vi "vector space.vi"(10 "Full transition sequence from service to end":string[](array[string])=["0 1 0", "0 -1 0", "0 2 0", "0 4 0", "-4 1 0", "0 -4 0", "0 -2 0", "1 0 4", "1 -4 0", "0 -3 3", "0 -3 0", "1 -1 0", "-2 2 0", "0 1 -4", "2 0 -3", "0 -3 3 0", "-1 0 -1", "0 -1 1", "2 -1 0", "0 2 -1", "-3 0 1", "0 1 0 4", "1 0 4 0", "-3 3 0", "1 0 -3", "3 -2 0", "2 0 -3 0", "1 0 -1", "-4 0 -1", "0 -4 1", "2 0 -1", "0 -2 2", "-4 0 -3", "0 -1 1 0", "0 2 0 -3", "3 -3 0", "-4 0 1 0", "-4 1 -4 0", "-4 1 0 4", "0 1 -4 0", "-4 1 -4", "0 2 -1 0", "1 0 3", "0 -3 4 0", "-2 0 2", "1 0 1", "4 0 2 0", "0 2 0 3", "0 -1 2", "-1 0 -4", "1 0 -4", "0 -1 0 -1", "-1 0 2", "-1 0 -1 0", "1 0 -2", "0 -4 0 -1", "0 -2 2 0", "-1 0 1", "2 0 2", "0 1 -1 0", "0 3 -3 0", "-4 0 -2", "0 4 -4", "0 -4 0 -3", "0 4 0 1", "0 -2 0 2", "0 4 0 2 0", "-3 0 1 -4 0 -3", "2 0 1 0", "-2 0 2 0", "0 3 -2 0", "-3 3 0 -2 0", "3 -3 0 1", "-3 0 1 0", "4 -4 0", "0 4 -4 0", "0 -3 3 0 -2", "2 0 2 0", "-2 0 -1", "0 -4 0 1 0", "2 0 -4 0", "2 0 -1 0", "-1 3 -2", "2 0 1", "1 0 -3 3 0", "-4 1 -1", "-4 1 -1 0", "-1 0 -3", "3 -2 2", "-1 1 -1 0", "2 0 4", "1 0 -1 0", "0 -1 2 -1", "0 2 0 -2", "-3 0 -4 1", "0 1 0 -1", "-1 3 0", "0 -1 0 -4", "-2 0 -1 0", "4 0 4", "-4 1 0 4 0", "-4 0 -2 0", "-4 0 2", "0 -2 0 2 0", "0 2 0 -4 0", "2 0 4 0", "4 0 -2", "0 1 0 -4 0", "3 0 1", "2 -2 0", "4 0 -2 0", "0 2 0 4", "1 -4 0 1 0", "0 2 0 -2 0", "-2 2 0 -1 0", "-2 2 0 -1", "-1 0 4 0", "-2 0 4", "-4 1 0 3", "0 -3 0 1", "-2 2 0 -3 0", "0 1 0 3", "0 2 0 1", "0 1 0 1 -4", "0 1 -4 1", "-4 1 0 -3", "1 0 -3 0", "-3 0 -2", "2 -1 0 -1 0", "-3 3 0 -2", "1 0 4 -4 0", "0 -4 0 -3 0", "0 -4 0 1 0 -3 3 0", "0 -3 3 0 2 0 -3 0", "0 -3 3 -3 0", "3 -2 0 1", "-4 0 3", "-2 0 1", "0 3 0", "0 -3 4", "-3 4 0", "-3 0 4", "0 3 -3 0 1 -4 0 -3 3", "0 -2 0 -1", "-4 1 0 -2", "-4 0 -2 0 -1", "-2 0 -4", "0 1 0 -2", "0 -1 0 2 0", "0 -2 2 0 -1", "0 -3 -1 3", "-4 -1 0", "0 -1 2 0", "0 -3 0 -4", "2 0 -3 0 -4", "3 0 -1 1", "-4 1 0 -1", "-1 0 -1 2", "-1 0 -4 0", "0 -4 1 -1", "-3 3 -2", "2 -1 1", "4 -3 0", "1 -4 4", "0 2 0 -1", "1 0 1 0", "4 1 0", "0 2 0 2 0", "-4 0 -1 -3", "1 -4 0 -1", "0 -4 1 -4", "-1 3 0 -4 1 -4", "2 -1 3", "1 -3 0", "-2 0 1 -4", "1 0 -1 1", "0 -3 0 -4 1", "0 2 -1 0 1 -4", "0 -1 3", "0 -4 0 -1 0", "0 4 0 -2", "0 -2 0 -1 0", "0 -3 3 0 -2 0", "0 1 -1 0 -1", "0 -1 0 1 -1 0", "-1 3 -2 2", "-2 2 0 1 0 -1", "0 1 -1", "0 4 0 1 0 4", "-3 0 -4", "1 0 4 0 4 0", "4 -4 0 -2", "4 0 2", "-1 2 0", "1 -1 0 -1", "4 0 1", "2 0 3", "0 2 0", "0 -1 0", "0 1 0", "0 3 0", "0 -4 0", "-2 2 0", "1 -1 0", "0 -2 0", "0 -1 2", "0 1 -1", "0 3 -2", "3 -2 0", "0 2 -2", "-1 0 3", "2 -1 0", "-1 0 -1", "-1 0 -3", "-2 2 -2", "2 0 1", "2 0 2", "0 -3 0", "3 -2 2", "0 1 -1 0", "0 -2 2", "-1 2 0", "2 0 -1", "2 -2 0", "3 -3 0", "0 -1 2 0", "0 -1 0 3", "0 -1 1", "0 2 0 1", "2 -2 2", "0 -4 4", "0 4 0", "2 0 3", "-2 3 -2", "2 -2 3", "4 -4 0", "0 1 0 -3", "0 3 0 3", "-1 0 4", "-3 0 -2", "-4 0 -2", "2 0 2 -1", "-1 0 2", "-2 0 -1", "-4 4 0", "0 2 0 -2", "-1 1 -1", "-1 1 -1 0", "-2 0 -2", "3 0 -4 0", "3 0 3", "0 1 0 3", "0 3 -3 0", "2 0 -2", "3 0 -2", "0 -3 3", "3 -2 2 -2", "-3 0 -2 0", "1 0 -3 0", "-1 0 2 0", "3 0 -4", "-1 0 1", "-1 0 -1 0", "0 -1 2 3", "-1 3 -2 0", "3 -1 3", "-2 0 2 0", "0 1 0 -3 0", "0 -4 0 -2", "1 4 -4", "0 -2 2 0", "1 4 0", "0 3 -2 0", "-2 0 -4 4", "-1 0 3 0", "0 2 0 -1", "0 2 -2 3", "4 0 -1", "-1 2 0 2", "1 -1 0 -3", "-2 0 2", "2 0 -4", "0 3 -2 2 -2 2", "0 2 -2 0", "4 0 -4 0", "0 3 0 3 0", "4 -3 0", "-3 4 -3 0", "0 4 -4", "3 0 -1", "-2 2 -2 0", "0 -2 3", "-2 0 3", "1 0 -3", "2 -2 2 0", "0 -3 4", "0 -1 1 -1", "0 4 1 4", "1 -1 0 -1", "1 4 -4 0", "-4 0 2 0", "-4 0 2", "0 -2 2 3 0", "0 -1 1 -1 0", "0 2 0 1 4", "4 0 1 0", "2 3 -2", "0 -1 2 3 -2", "0 -1 0 4", "-4 0 1", "-1 0 -1 2", "-2 0 -1 0", "0 3 0 -1", "3 -2 0 -1", "0 -4 0 -2 0", "2 0 -4 0", "0 -2 0 2", "-1 0 -3 0", "0 -3 0 -2", "2 0 -1 0", "0 -1 2 0 1", "0 -2 0 -4 4 0", "0 -4 4 0", "-1 -3 0", "0 -2 0 3", "2 0 -2 2", "-4 1 0", "-1 1 4", "-1 0 3 -2", "0 2 0 4", "0 -4 4 0 -1", "3 0 -2 0", "0 3 0 -2", "2 0 1 -1 0", "0 1 -1 0 2 0", "0 2 0 1 -1", "2 0 -1 2", "-2 3 0", "0 -1 0 2", "0 1 -1 0 -3", "2 0 1 -1", "-2 0 -1 2", "-1 4 0", "0 -4 1", "2 0 2 0", "2 -1 1", "4 -4 0 -1", "-4 0 -1", "-1 0 4 0", "2 0 2 -1 0", "0 -3 3 0", "-1 0 -3 3", "-1 0 1 -1 0", "0 3 0 -4", "-2 2 -2 0 -2", "-2 0 4 0", "0 1 0 3 0", "4 -3 0 -2 0", "0 3 -2 3", "2 0 3 -2", "3 -2 3", "0 2 -2 3 -2 2", "-2 2 0 3", "3 -2 2 0", "3 -2 2 0 3", "3 -2 3 -2", "0 -3 4 -3 0", "0 -1 0 -3", "3 -3 0 1 0", "0 2 0 3", "0 3 -2 2 -2 2 0", "0 2 0 2", "-2 3 -2 0", "4 0 -2", "-4 0 -1 0 3", "-2 2 -2 3", "0 -1 0 -1 0", "-2 2 0 3 0", "0 2 -2 2", "2 3 -2 2 0", "-2 2 -1", "-4 0 -2 2", "0 -4 0 2", "-1 2 -1", "-1 0 3 -1 3 0 -4", "-1 3 -2", "4 0 -4", "3 0 3 0", "0 3 0", "0 1 0", "0 2 0", "0 4 0", "0 4 -4", "0 -3 4", "0 -3 0", "0 -4 0", "0 3 -2", "0 -1 0", "-4 1 0", "1 0 3", "0 2 0 -3", "2 0 3", "3 -3 0", "-3 0 3", "0 -3 3", "0 -3 4 -3 0", "0 -2 0", "3 -2 0", "0 3 0 1 0", "0 -3 4 0", "2 -2 0", "-2 0 -3", "4 0 2", "-3 0 2", "0 3 -3 0", "4 -4 0", "0 -1 2", "3 0 4", "0 3 -2 0", "0 -3 0 3", "1 0 -1", "0 4 -4 0", "-2 0 3", "0 2 -2 0", "0 2 0 -3 4", "3 -3 0 -3", "4 0 2 0", "3 0 -2", "0 -3 3 0", "-1 0 3", "0 -1 2 0", "-4 0 -1", "2 0 3 0", "0 3 0 3", "-4 0 3", "0 4 -4 1", "4 0 -3", "0 -1 0 4", "0 3 -3 0 2", "0 -2 0 3", "0 -3 4 0 3 0", "-3 0 4 0", "0 3 0 3 0", "0 4 0 -3 0", "-3 4 0", "2 0 -3 4", "0 2 0 -3 4 0", "0 1 0 2", "0 -2 3", "-2 0 -2", "0 -3 4 0 2", "0 -3 3 0 -2 2", "1 0 -3", "0 -1 1 0", "4 -4 0 -4", "-4 0 3 0", "2 0 -3", "-2 0 3 0", "0 4 -4 1 0", "-4 1 0 -1 2 0", "3 0 4 -4", "0 -3 4 -3 0 2", "3 0 3", "-1 0 -3", "-3 4 -3", "4 -3 0", "0 -3 4 -3", "-3 4 -3 0", "4 0 2 0 3", "0 2 0 3", "-4 1 0 -4 0 4 -4", "-4 1 -1", "-1 0 -4 0", "1 0 3 -2", "0 -1 0 3", "0 3 0 4 0", "0 2 0 3 0 1 0", "-4 1 -4 1", "1 -4 1 0", "0 -4 4", "0 1 0 4", "1 -4 1", "-3 0 1", "0 4 -4 0 -1 0", "-3 0 4", "2 0 -3 4 0", "1 0 2", "4 -3 0 2", "-3 4 -3 0 2", "3 0 1", "1 -1 0", "0 -1 0", "0 1 0", "0 1 -1 0", "0 4 0", "0 3 0", "-1 0 4", "-1 0 -3 3", "1 0 1", "-4 1 -1", "0 4 0 2", "0 -1 0 -3", "3 -2 2 -1 0", "2 -1 0", "0 1 -1", "-1 0 3", "-1 1 -1 0", "-3 0 1", "-1 0 3 0 -4", "-1 0 -3", "1 -1 0 -3 3", "1 -1 0 3", "2 -1 0 4 -4", "1 0 1 0", "0 -1 0 4", "2 0 3 0 -1", "-4 1 -1 0", "0 3 0", "0 -1 0", "0 4 0", "-1 0 3", "0 -3 4", "0 -3 3", "1 -1 0", "0 3 -2", "0 2 0", "0 1 -1", "4 -3 0", "-4 0 -3", "0 -4 0", "4 0 2", "0 1 -1 0", "0 1 0", "0 4 -4", "3 -2 2", "2 -1 0", "0 -2 0", "0 -3 4 0", "-1 0 -3", "0 3 -2 0", "0 -3 3 -3 0", "0 -3 4 -3 0", "4 0 4", "0 1 -1 0 3", "3 -2 2 0", "-2 2 0", "3 0 1", "0 4 0 2", "0 2 -1", "2 0 4", "-1 0 4", "0 -3 3 0", "-1 0 1", "-1 0 -1 0", "-1 0 -1", "4 -3 0 2", "0 -3 0", "-4 0 -3 0", "-3 0 3 -2", "0 3 -2 2 0", "-4 0 -3 3", "0 3 0 -4", "2 0 4 -4", "0 2 0 4", "0 4 0 -4", "2 -1 0 1 -1 0", "0 2 -1 0", "-1 0 -3 3", "0 -4 4 0", "0 4 -4 0", "-4 0 3 0", "0 -2 3", "-3 0 -3", "0 -2 0 -3", "-3 0 1", "-2 3 0", "0 3 0 -2", "0 4 -3 0", "4 -3 0 2 0", "0 -3 4 -3 0 3 -2 2 0", "3 0 -3 4 -3 0", "-1 0 3 -2 3", "-1 0 3 -2", "0 1 0 3", "1 0 3", "4 -3 0 -2", "-4 0 -3 4", "-2 0 3 0", "2 0 2", "0 2 0 2 0", "-4 4 -3 0", "0 -4 0 -3", "3 0 3 0", "-4 0 -3 3 0", "4 0 3", "0 4 0 4", "4 0 4 0", "0 4 0 -4 0", "0 -1 0 -2", "4 0 2 0", "1 0 -3", "0 -4 1 -4", "0 4 -4 0 -3", "-2 2 0 4 -4", "0 4 -4 4 -4", "4 0 2 -2", "0 4 0 -2", "0 3 0 1", "4 -4 1", "4 0 2 -1 0", "0 -4 4 0 2", "-1 0 3 0", "0 3 -2 0 -1 0", "1 -1 0 4", "0 4 0 1", "-1 0 4 0", "1 0 3 -2 0 -1 0", "0 -4 0 3 0 -4", "-1 0 -4", "1 -4 0", "1 0 4 0", "0 -1 0 -1 0", "-1 0 -3 3 0", "0 -1 0 -1 0 -3", "-2 2 -1 0", "0 -1 0 3 -2", "2 -1 0 1 -1 0 3", "-2 3 -2 2 -1", "-2 2 -1", "0 -1 0 4", "3 0 1 0", "0 3 -2 0 -1 0 -1 0", "-3 4 0", "3 0 -1", "0 4 -3", "3 0 3", "-4 0 3", "4 -4 0", "0 -1 0 -1", "0 3 0", "0 -3 4", "0 -3 3", "0 3 -3 0", "0 2 0", "4 -3 0", "0 3 -3", "0 3 -2", "0 -3 4 -3 0", "-4 0 -3", "3 0 -3", "0 -4 0", "-3 0 -3", "0 -3 3 0 3", "0 -3 3 0", "0 -2 0", "-3 0 3", "3 -3 0", "3 0 3", "-3 4 0", "-4 0 -3 4", "-3 0 4", "0 -1 0", "3 0 -3 3", "-3 3 0", "0 3 -2 0", "0 -3 4 0", "1 0 -3 4", "0 -3 0", "0 -1 0 -3", "-3 0 3 0", "-2 0 3 -2", "0 1 0", "0 -2 0 3", "-2 0 -3", "0 3 0 -3", "3 0 3 -3", "3 -3 0 3", "-3 0 -3 3 0", "0 -3 4 -4 0", "0 2 0 -2", "-2 0 3", "0 3 -2 3 0", "-2 3 0 -3 3", "3 0 -1", "-3 0 -4", "1 -1 0", "-4 0 -2", "0 3 -3 0 4", "-2 3 0", "-1 0 3 -2", "-3 4 -3", "0 -3 4 -3", "-3 4 -3 0", "-3 3 0 3", "-2 0 2", "0 -1 0", "0 -2 3", "3 -2 0", "-2 3 -2 0", "0 2 0", "0 1 0", "0 4 0", "2 0 -1 0", "0 3 -2", "2 -2 3", "-2 0 2", "0 2 -2 0", "4 -3 0", "-3 0 -2 0", "0 3 0", "0 -3 -2", "-2 3 -2 0 3", "0 3 0", "0 -2 0", "0 1 0", "0 3 -2", "2 -2 0", "0 2 0", "3 -2 0", "0 -3 4", "0 4 0", "-2 0 -2", "0 -3 0", "3 -2 2", "1 -1 0", "0 2 -2", "-2 3 -2", "0 -1 0", "0 -4 0", "0 2 -2 0", "-1 0 3", "0 -2 3", "2 0 -2", "0 3 -2 0", "0 -3 4 0", "-3 0 3", "0 3 -3", "4 -3 0", "-2 0 -3", "0 -2 3 -2", "-2 2 0", "0 3 -2 2", "3 -2 2 0", "2 0 2", "3 -3 0", "2 0 3", "0 -2 0 -2", "-3 4 0", "0 3 -3 0", "-1 0 3 0", "-2 0 1", "2 -1 0", "0 -3 4 -3", "0 3 -2 2 0", "-2 0 1 0", "-3 0 4", "0 -2 2", "-2 3 -2 0", "0 3 -2 3", "0 1 -1 0", "1 0 1", "0 -3 0 3", "0 -3 3", "3 0 -3", "0 -1 0 3", "4 0 1 0", "0 -2 3 -2 0", "2 0 3 -2 0", "0 2 -1", "3 -3 0 4 0", "-2 0 -4", "-3 0 -2", "3 0 3", "0 3 0 3 0", "0 3 -2 3 -2", "-2 3 -2 2", "-3 0 1", "-2 0 3", "-2 0 -3 0", "0 3 -2 2 0 2", "2 0 2 0", "1 -1 0 3", "0 3 -2 0 -2 2", "-2 0 -2 2", "2 0 -2 3 -2", "1 0 -2", "1 0 3", "2 0 -4 0", "-1 0 1", "0 2 0 4", "4 0 -2", "0 -2 0 1", "0 -1 0 3 0", "0 2 0 3 -2 0", "0 3 -2 0 1 0", "-1 0 -1 0", "-2 2 0 -2", "2 0 -2 0 -2", "0 4 0 1 0", "0 1 0 4 0", "0 1 0 -3", "0 -3 0 3 -2", "1 0 -3 0", "4 0 -4 0 1", "-1 0 -4", "0 -3 3 -3 0 4 0", "0 -4 0 3", "0 3 0 2", "1 0 1 0", "0 4 0 3", "1 -1 0 -3 4 0", "3 -2 0 -4", "2 -1 2 0", "-4 1 0", "3 -2 0 -4 0", "-2 0 -3 4", "0 -3 4 -3 0", "0 -2 0 -3", "-2 0 -3 4 -3 0", "2 -2 3", "0 2 -1 0", "2 0 2 -2 0", "0 -3 4 0 2", "1 0 2", "-3 4 0 2 0", "-2 0 -4 1", "0 3 -2 0 -4", "0 2 0 2", "-2 3 0", "1 0 -3", "0 3 0 -3 4", "-3 4 0 2", "-2 0 -2 2 -2 0", "2 -2 0 -3 4", "0 -3 4 -3 0 3", "4 -3 0 3 0", "3 0 -2", "0 -2 0 -2 0", "4 -3 0 3", "0 4 -3 0", "-3 0 -2 0", "-1 0 -1", "1 0 4", "2 0 2 -2", "-2 0 -2 0", "1 -1 0", "-1 0 1", "0 1 0", "0 -1 0", "0 1 -1", "-1 0 -1", "0 4 0", "2 -1 0", "-1 0 1 -1", "-1 0 4", "0 -3 0", "0 1 -1 0", "-1 1 -1", "-1 0 -3", "-1 0 -1 0", "0 -1 0 1", "1 -1 0 -1", "-1 1 -1 0", "1 -1 1", "4 0 2", "0 1 -1 0 1", "1 -1 0 4", "0 1 0 -4", "0 4 -4", "-1 0 -1 0 1", "-1 0 4 0", "0 1 -1 1 -1 0", "1 0 -4 0", "1 0 -4", "0 4 0 -1 0", "-1 0 1 0", "0 4 -4 0", "-1 0 -3 4 0", "0 1 0 -1 0 -3", "0 1 0 -4 0", "-4 0 4", "0 -1 1 -1", "-2 2 -1 0", "0 -3 0 -1 0", "2 -1 0 -3", "-1 0 3 0", "-1 0 -3 0", "-1 0 -2", "0 2 0", "1 -1 0 4 0", "-1 0 4 0 -1 0", "0 1 -1 1 -1 0 4", "0 -2 2 -2", "-1 0 -1 0 1 0", "3 0 1 0", "0 4 0 1 -1", "1 -1 0 1", "0 1 -1 1", "1 -1 1 -1", "0 1 -1 1 -1", "1 -1 1 -1 0", "0 -1 1", "0 -4 0", "-3 0 -1", "4 0 -1", "-1 1 -1 0 4", "1 -1 1 -1 0 4", "-2 2 0", "1 -1 0", "0 1 0", "0 -1 0", "3 -3 0", "0 3 0", "0 1 -1", "0 4 0", "0 2 0", "2 -1 0", "-1 0 1", "0 -2 0", "-4 1 0", "1 0 1", "0 1 -1 0", "-1 0 -3", "-1 0 4", "0 4 0 -2", "0 4 -4", "-1 0 1 0", "0 3 -3 0", "0 -4 1", "0 4 -4 1", "-4 4 0", "-1 0 3", "0 -2 3", "0 -3 4", "1 0 1 -1", "-2 0 -3", "0 -3 0", "0 -3 3", "-2 3 -3 0", "1 0 -2", "-2 3 -2", "4 -4 1", "1 -1 0 4 -4 1", "-1 0 4 -4 1 -1", "-4 1 0 1 -1 0", "0 1 0 -4", "0 1 0 -2", "-1 0 -1 0", "2 -1 0 1", "1 -1 0 1 0", "3 -2 0", "0 -2 2", "2 0 2", "3 -3 0 1", "-3 0 3", "-2 2 0 -3", "0 3 -3", "-3 0 -4 4", "0 4 0 -2 3", "0 -4 4", "-1 0 3 0", "4 -4 1 0 4", "4 0 1 0", "1 -1 0 -3", "-2 0 1 -1", "0 4 -4 1 0", "0 -4 4 0 1", "1 0 -2 3 -2", "1 0 4", "0 -4 1 0", "0 1 0 -4 1 0", "-2 0 1", "4 -3 0", "-3 0 4", "0 4 -3 0", "1 -1 0 4 -4 1 -1 0", "4 -4 1 0", "1 0 4 0", "1 -1 0 -1 0", "0 -4 0", "4 0 1", "0 1 0 1 0", "2 0 4 0", "0 -2 0 2 0", "2 0 1", "-1 0 -3 4", "4 0 2 0", "0 -2 0 1", "-1 0 4 -4 1", "3 -2 3", "3 -2 2 0", "1 -1 0 3", "-1 0 -1", "0 -1 1", "-1 0 1 0 3", "0 -4 1 0 1 -1 0", "0 3 -2", "0 1 0 3", "1 -4 0", "0 -2 2 0", "1 -1 1 -1 0", "0 1 0 3 -3 0", "-3 0 -3 3", "0 -3 3 0", "0 3 0 -2 0", "0 2 0 2", "-4 0 -2", "3 0 3", "3 0 3 0", "0 -3 3 -2", "0 2 -2 3 -3 0", "-2 2 0 -3 3", "-3 0 1", "3 -3 0 3", "0 3 -3 0 1", "0 3 0 2", "2 0 -3", "-2 3 -3", "3 -2 2", "-4 1 -1", "2 0 -3 3", "0 4 0", "0 -2 0", "1 -1 0", "-1 2 -1", "0 2 0", "2 -1 0", "0 3 0", "0 -1 0", "-2 0 3", "0 -4 0", "3 -2 0", "0 3 -2", "0 -3 0", "-1 0 3", "0 -2 0 3", "0 1 -1 0", "0 3 -2 0", "1 -4 0", "-1 0 2", "0 -1 2", "2 0 3", "0 -3 3", "3 -3 0", "3 0 -1 0", "-2 0 -2", "2 -2 0", "-3 3 0", "0 2 0 3", "0 1 0", "0 -2 2", "-4 0 -1", "0 -1 2 -1", "-1 0 -1", "2 -1 2", "-1 3 -2", "3 0 -4", "3 -2 2", "-1 1 -1 0", "-1 2 -1 0", "0 1 -4", "4 -4 0", "2 -3 0", "0 3 0 -2", "2 0 3 0", "0 1 0 -3", "1 0 -3", "-1 0 -4 0", "-4 0 1", "2 0 -2 0", "-1 0 -3", "0 -3 4", "4 0 1", "0 1 -4 0", "0 -1 0 3", "0 -3 3 0", "0 3 -3 0", "0 4 0 2", "0 2 -2 0", "-2 0 -3", "3 0 3", "-1 0 -2", "-2 0 3 0", "2 0 4 0", "0 4 0 -2 3", "0 -3 0 -2", "-3 0 -2 2", "1 0 4 0", "-3 0 2", "0 -2 0 3 -2 0", "1 0 -3 0", "-3 0 -2", "-2 0 -2 0", "0 4 -4", "-1 -3 0", "-2 2 -1", "2 0 -3", "-1 1 0", "2 -1 1", "-2 2 0", "0 -4 0 -1", "0 -1 3 -2 2", "-1 2 -1 2", "-1 2 0", "-1 3 0 -1 0", "2 0 2", "-1 0 2 -3 0", "-1 0 2 0", "-1 4 -4 1", "-1 0 4", "2 -1 0 -1", "2 -1 0 2", "-4 1 -1", "3 0 -4 1", "1 -1 -3 3", "0 1 0", "0 -2 0", "1 -1 0", "0 3 0", "0 2 0", "0 3 -2", "3 -2 0", "0 -4 0", "-1 0 -2", "-2 2 0", "0 -1 0", "1 -1 0 -2", "0 -2 2", "-2 0 -2", "0 1 0 1", "4 -4 0", "0 3 -3", "0 1 -1", "1 0 1", "0 3 -2 0", "-2 2 -2", "0 -2 3", "0 3 -3 0", "0 4 0", "2 0 3", "0 -2 3 -2", "0 4 -4 0", "-2 0 -2 0", "1 -1 0 -2 0", "-2 0 2", "-4 0 -4", "0 -4 0 1", "0 2 0 -4", "3 0 -2", "-1 0 3", "0 1 -1 0", "-3 0 -1", "-1 0 2 0", "4 -3 0", "1 0 -2", "0 1 0 1 0", "0 -2 3 -2 0", "3 -2 0 -2 0", "0 -2 2 -2 0", "0 -2 0 -2", "-1 4 0", "4 0 2", "1 -1 0 -2 0 2 0", "2 0 -2", "-2 0 4", "0 -1 0 3", "0 -2 2 0", "1 0 3", "0 1 0 3", "4 0 -2", "0 -4 0 -4", "0 2 0 -4 0", "-4 0 -4 0 1 0", "-1 2 3 0", "3 0 3", "0 -4 0 3 0", "2 0 1", "2 -1 0", "-1 0 -1", "-2 3 0 -2", "3 0 -2 0", "0 1 -1 0 -2", "0 3 0 -2", "3 -2 2 -2", "1 0 1 -1", "0 4 -3 0", "2 0 -1 0", "0 2 0 3", "2 0 3 0", "2 0 -3 4 -3", "-2 2 0 -3 4", "2 0 -3 4", "0 3 -3 0 -1 0", "1 0 4", "0 3 0 1", "1 0 3 -2 0", "-2 3 0", "1 0 1 0", "0 4 0", "0 2 0", "0 3 0", "0 -3 0", "0 1 0", "-4 0 -3", "0 -4 0", "0 3 -3 0", "0 -3 0 3", "-4 0 3", "0 4 0 2", "0 -3 3", "-4 0 -3 0 3", "0 2 0 3", "-3 0 2", "0 4 0 1", "0 -4 0 3", "0 4 0 2 0", "0 -2 0", "0 1 0 4", "4 0 2", "0 4 0", "0 3 0", "0 2 0", "4 -4 0", "0 4 -4 0", "0 -2 0", "3 -3 0", "0 4 -4", "0 3 -3", "0 3 -2", "0 4 0 2", "4 0 2", "0 1 0", "0 3 -3 0", "0 -3 0", "2 -1 0", "0 -1 0", "1 0 3", "4 0 3", "3 -2 0", "0 1 -4", "-1 0 4", "0 -4 0", "0 -3 3", "2 0 4", "-4 1 0", "0 -2 2", "0 4 0 3", "-1 0 1", "0 3 -2 0", "-3 0 4", "-1 0 3", "0 -3 4", "0 4 0 -2", "1 -1 0", "2 0 4 0", "0 -4 4", "0 -1 0 4", "-1 0 4 0", "4 -3 0", "0 2 -1 0", "1 -4 0", "2 0 -4", "-2 0 4", "0 4 0 2 0", "3 0 3", "0 -3 3 0", "2 -2 0", "1 0 -3", "-4 0 2", "1 0 3 0", "0 1 0 3", "-1 0 3 0", "3 -2 2", "-4 1 -1", "2 0 -3", "0 -4 1", "0 2 0 -4", "-3 0 4 0", "3 0 -2", "0 -2 2 0", "0 -2 3", "-4 0 2 0", "0 3 0 -4", "0 2 0 4 0", "-2 0 2", "-2 2 0", "0 3 0 4", "-3 4 0", "-1 0 1 0", "4 0 4", "0 1 0 3 0", "0 -1 0 4 0", "0 3 0 3", "1 0 -3 0", "0 3 0 1", "-2 2 -1 0", "0 3 -2 2", "-3 0 2", "1 -1 0 3 0", "0 3 0 -2", "-4 0 -4", "0 1 0 -3 0", "0 4 0 -3", "2 -1 0 4", "1 -4 1", "-4 0 3", "-2 0 -4 0", "0 3 -3 0 4", "-4 0 -2", "0 4 -4 0 3", "0 -2 3 -2 0", "0 4 0 4", "-1 2 -1", "-3 0 -2", "-3 0 -3", "-4 0 4", "4 0 -3", "3 0 -4", "2 0 -2", "-2 0 2 0", "0 -4 4 0", "0 2 0 3", "-2 0 1", "4 0 3 -3 0", "0 -2 0 3", "0 4 0 3 0", "0 2 -2 0", "2 -2 0 4", "4 0 -2", "2 0 -1", "0 1 -4 0", "0 -1 2", "4 0 -1", "0 1 -4 1", "4 -4 1", "0 3 -2 0 1", "4 0 4 0", "0 -1 0 4 0 4", "1 0 4", "0 1 -4 1 0", "0 4 0 2 0 -3", "-2 0 4 0", "0 2 -2 0 4 0", "0 -3 0 2", "-4 0 -2 0", "0 -2 0 2 0", "0 2 0 -1", "0 -1 3", "0 -4 4 -4", "3 -2 0 -4 0", "-4 0 -1", "-3 0 3 0 3", "-1 0 3 -3 0", "-3 0 3 0", "0 3 0 3 -2", "-2 2 -2", "-1 0 1 0 3", "-2 2 -1 0 1 0", "0 2 -1 0 -3", "0 4 0 2 -1 0", "-1 0 4 -4 0", "0 2 -1 0 4 -4", "0 4 -4 0 3 -2 0", "-1 0 -3", "-2 0 1 -4", "0 3 0 4 0", "0 1 -4 4", "-1 0 -3 0", "-1 0 4 -4", "0 4 0 -2 0", "0 4 -3 0", "4 0 -3 3", "-1 0 -2", "0 -2 0 3 -3", "1 -4 1 -1 0", "-4 1 -1 0", "-2 0 -2 2", "0 -1 2 -1", "-4 0 -4 1", "0 2 0 4 0 2 0", "0 3 0 -1", "3 0 3 0", "0 -3 0 3 0", "0 3 0 4 -4 1", "-1 0 -4", "0 -4 1 0 3 0", "0 2 -1", "-4 0 4 0", "0 -2 0 4", "0 4 0 -1", "-4 0 3 0", "0 3 0 -2 0", "0 -3 4 -3 0", "-4 0 2 0 -4", "2 0 -2 0", "-2 2 0 -3", "3 0 2 0 4 0", "3 0 2 0", "1 -4 0 2 0", "3 0 -4 4 0", "3 0 -4 4", "3 -3 0 4", "-2 3 -3", "0 -4 0 2 0", "0 3 0 -4 0", "3 -3 0 4 0", "0 3 -3 0 4 0", "4 0 3 -2", "-4 0 -3", "-3 0 -3 4", "3 -3 4 0", "1 -4 -1", "-3 3 -3 0", "0 -1 1", "-3 0 4 0 3", "0 3 -3 0 -2", "0 4 0 3 -3 0", "4 -3 0 4", "0 3 0 2 0", "0 4 0 -2 2", "-4 -1 0 1", "-1 0 1 0 -3 0", "-3 0 1 -4 0", "-3 3 0", "0 -1 0 1", "-1 0 1 -4", "0 3 0 -4 4", "-4 1 -1 0 3 0", "0 1 0 3 0 1", "-3 0 3", "4 0 -2 0", "4 0 2 0", "3 0 -1", "4 0 3 -3", "3 -3 0 -2", "3 0 4", "3 0 2", "2 0 3", "4 0 -2 2", "-2 2 -1", "0 2 -1", "0 4 0", "2 -1 0", "0 -4 0", "0 2 -1 0", "3 -2 0", "4 -3 0", "0 -1 2 0", "0 -1 0", "0 2 -2", "-4 0 1", "-4 0 -4", "0 -4 0 -4 0", "-1 0 4 0 2", "-2 2 0", "1 0 -4 0", "3 -2 2", "0 2 3 -2", "2 -1 0 2 -1", "2 -1 -3", "3 -2 0 -4", "0 -3 4 -3 0", "-1 1 -1 0 -1", "0 -4 1 0", "-1 0 2", "4 0 2", "0 2 0", "0 1 0", "0 -4 0", "0 -2 0", "0 2 -2", "2 -2 0", "0 4 0", "0 3 0", "0 2 -2 0", "0 -1 0", "0 -3 0", "-4 0 -2", "-2 0 2", "1 0 4", "-2 0 -4", "0 3 -2", "3 -2 0", "1 -1 0", "-2 3 0", "0 -1 2", "0 -3 4", "4 -3 0", "-2 0 4", "0 4 -3", "-2 0 -4 0", "-2 2 -2", "3 0 1", "4 0 2", "-1 0 -1", "0 -2 3", "1 0 -4", "-1 0 -1 0", "-2 0 -3", "1 0 -3", "-2 0 3", "2 0 -2", "-2 2 -2 0", "-4 0 -2 0", "0 1 0 4", "0 3 -3", "2 0 1", "1 -4 0", "0 -4 1", "0 3 -2 0", "-3 4 0", "0 -4 0 -2", "2 -1 0", "0 3 0 1", "0 1 -4 0", "3 0 2", "-3 0 -4", "-4 0 2 -2 0", "0 -4 0 2 -2", "2 0 -2 0", "0 4 -3 0", "-4 0 2", "-4 0 2 -2", "-2 2 0", "-4 1 0", "0 4 -4", "-2 0 2 0", "0 -2 0 2", "1 0 3", "-2 0 4 0", "2 0 -4", "-2 3 -2", "0 2 0 1", "0 4 0 2", "0 2 -2 2", "0 1 -1", "0 -4 0 -3", "-1 0 -4", "-1 0 -2", "2 -2 0 -4 0", "2 0 3", "0 -4 0 2", "0 -3 4 0", "0 3 -3 0", "0 -4 0 -2 0", "-2 0 -2", "0 -3 3", "0 -2 0 -4", "0 -4 1 0", "4 0 2 -2", "-3 0 -4 0", "0 -3 4 -3 0", "2 -2 0 2", "0 1 0 -1", "2 -2 0 4 0", "2 -2 0 4", "1 0 -4 0", "-3 0 3 0", "0 3 0 -2", "2 -2 3", "0 2 0 -2 0", "0 1 0 3", "1 0 4 0", "-4 4 -4 0", "-2 0 1", "0 -4 0 3 0", "1 0 1 0", "-1 0 3", "0 -1 2 -1", "0 -1 0 -1", "0 4 0 3", "0 -2 0 4", "0 -4 4", "0 3 0 1 0", "1 0 -3 3", "0 2 -1", "-1 0 1", "-2 0 -3 0", "1 -1 0 -2", "-1 0 -2 0", "3 0 3", "-1 1 0", "3 0 -2", "3 0 4 0", "0 2 -2 2 -2 0", "0 1 0 -4", "0 2 0 4 -3", "-2 0 -2 0", "0 3 0 -2 0", "-2 0 -2 3", "0 2 0 3", "0 -2 0 2 0", "0 -3 3 0", "4 0 -3", "0 1 0 -3", "1 0 4 -3 0", "2 -2 0 -2", "0 -1 1", "-1 1 -1 0", "0 1 0 -1 1", "0 -3 0 -3", "-1 0 -3", "4 -3 0 1", "-3 4 0 2", "0 2 -2 0 -3 4", "3 -2 0 -3 0", "0 -2 0 3", "-2 0 -4 0 2", "0 2 -2 0 -4 0", "0 -2 0 4 0 3", "4 0 -2 0", "0 -4 0 -3 4", "0 1 0 -4 0", "0 -2 2", "0 4 0 4", "2 0 -4 0", "-4 0 -1 2", "3 0 3 0", "0 3 0 2", "0 2 -1 0", "2 -2 3 0", "0 1 -1 0", "0 1 0 4 0", "0 1 -4 0 -2", "0 -2 0 2 -2 0", "0 -2 0 -3", "-4 0 1", "-2 0 2 -2 0 3 0", "-2 0 3 0 1 -4 0", "4 -1 0", "0 2 -2 0 2", "2 0 2 -2", "1 0 -4 4", "-1 0 4", "2 -1 0 -4 0 -3", "0 -1 2 -1 0", "-1 0 3 0", "-3 0 3 0 1 0", "1 -4 0 -4", "0 1 0 -2", "-2 0 -4 0 3 0", "0 4 0 2 -2 2 -2 0 -4 0 3", "0 2 -2 0 4", "-2 0 2 -2 0", "0 -1 1 0", "1 -1 0 -2 0", "0 -4 0 3", "4 0 1", "-2 0 -1", "-1 0 -1 0 -1", "0 1 0 3 0", "-1 2 0", "-1 0 1 0", "3 -2 3", "0 -2 3 0", "3 0 2 0", "0 3 0 4 0", "-1 0 2", "0 -3 0 -1 0", "-4 0 -3", "-1 0 -2 3", "0 -2 3 -2", "0 -2 3 -2 0", "-2 0 -4 0 3", "0 3 0 3", "0 -2 0 -4 0", "0 4 0 -4 0", "1 0 2", "3 0 -2 3 -2", "-3 0 2 -2 0", "4 -3 0 2", "-3 0 -2 0", "2 0 4", "0 2 0 4", "2 0 4 -3", "0 2 0 4 -3 0", "-3 0 2", "-3 0 -3", "4 0 4", "1 0 -2", "-2 0 2 -2", "1 0 1", "2 0 4 -3 0", "-3 0 3", "3 -3 0", "0 3 0", "-3 3 -3 0", "-3 3 -3", "0 -3 3 -3", "0 -3 3 -3 0", "2 -1 0", "0 -3 3", "-3 0 -3", "3 -3 0 -3", "-3 0 -3 3", "0 2 -1", "0 1 0", "0 3 0 3", "0 -1 0", "3 -3 0 -3 3", "0 2 -1 0", "0 4 0", "0 3 -2", "-1 0 2", "3 -2 0", "0 -4 0", "0 -3 0", "3 0 2", "0 3 -3", "0 -3 4", "-3 0 -3 3 -3", "0 3 -2 0", "-1 0 4", "-1 0 3", "-1 0 3 0", "0 1 0 3 0", "1 0 -1", "0 1 0 -1 0", "3 0 1", "0 2 0", "0 -1 2 0", "-3 0 -2", "3 0 -3", "0 -2 3", "0 -3 3 -3 0 -3 3", "3 0 3", "0 2 -1 0 2", "0 2 -2", "2 -2 3", "1 -1 0 3", "0 3 -2 0 1 0", "0 4 0 -1", "0 1 -4", "2 -1 0 4", "0 4 -4", "0 1 0 3 0 1 0", "1 0 3", "0 1 0 3", "1 0 3 0", "2 0 -1", "0 -1 0 3 0 3 0", "0 2 0 3 0", "2 0 4 0 2", "-4 0 -3", "4 -4 0", "0 3 0 3 -3", "-4 0 3 0", "0 -3 4 -3", "-3 3 0", "-2 0 3", "0 -2 0", "1 0 -3", "2 -2 0", "3 0 -3 4", "-3 0 -3 3 -3 0", "3 -3 0 -3 3 -3 0", "0 -3 3 -3 0 -3 3 -3 0", "0 3 0 -3", "-3 3 -3 0 -3", "0 -3 3 -3 0 -3", "-3 3 -3 0 -3 3", "2 -1 0 2", "3 0 3 0", "2 0 3", "3 -3 0 -3 3 -3", "0 3 0", "0 2 0", "0 4 0", "0 -3 4", "0 1 0", "2 -1 0", "0 -1 0", "0 -3 3", "2 0 3", "0 4 -4", "1 -1 0", "0 3 -2", "3 0 3", "0 2 -1", "-4 0 -3", "0 -3 0", "-1 0 4", "-1 0 2", "4 -4 1", "4 -4 0", "0 -2 3", "3 -3 0", "0 1 -1", "0 1 -4 0", "3 0 3 0", "1 -4 0", "0 2 0 3", "3 -2 0", "0 3 0 3", "-1 0 3", "1 -1 0 4", "0 2 -1 0", "0 -3 4 -4", "3 0 1", "0 -2 0", "0 4 -4 0", "0 3 0 3 0", "1 0 3 0", "3 -2 2", "-4 0 -3 3", "3 0 -3", "0 -3 3 -3 0", "3 0 -2", "-4 1 0", "0 -4 4", "2 -1 0 -3", "0 3 0 1", "2 0 -3", "-3 0 1", "-4 1 -1", "0 2 -2", "-2 3 0", "1 0 1", "0 -1 0 2", "0 3 -2 2", "0 1 0 3", "0 -4 1", "0 -3 3 0", "-2 2 0", "-2 0 3", "1 0 4 0", "4 -4 1 0", "0 1 -1 2", "1 0 1 0", "0 1 0 1", "-1 0 4 -4", "2 -1 0 3", "1 -1 2", "-1 2 -1 0", "0 4 -4 1 -1", "0 -3 4 -4 1", "4 -4 0 -3 3", "0 -4 4 -4", "-1 0 2 -1", "-2 0 -1", "1 -1 0 4 -4", "0 4 0 3", "2 0 4", "4 -4 0 -3", "0 3 0 -2", "0 -3 4 0", "1 0 3", "-4 0 3", "-3 0 2", "0 3 -2 3", "0 2 0 3 0", "0 4 0 2", "4 -3 0", "-3 0 1 0", "0 2 0 -3", "0 1 0 3 0", "0 -4 0", "0 -4 0 -3", "2 -2 0", "2 0 -2", "0 3 -3", "2 -1 0 -3 4", "-1 0 -2", "1 -1 0 3", "-1 0 3 0", "0 -1 2", "0 -3 4 -4 1 0", "0 4 0 -1", "1 0 -3", "0 3 -2 0", "0 1 0 4 0", "0 4 0 -4", "0 4 0 3 -2", "3 -2 0 1 0", "2 -1 0 -3 0", "-3 0 -4", "0 4 -4 1 -1 0", "-1 0 4 -4 0", "0 4 -4 0 2", "-3 0 -1", "0 3 0 1 -1", "-1 0 4 0", "0 1 -1 2 -1 0", "2 -1 0 2", "0 2 0 -1", "-1 0 -1 0", "-1 0 2 -1 0", "0 1 0 2", "0 2 0 -3 4 -4", "1 0 3 0 2", "0 -2 3 -2", "3 -2 0 -1", "0 4 -4 0 -3", "1 0 -4", "-4 0 -3 3 -3 0", "-2 3 -2 0", "-2 3 -2", "0 4 0 2 0", "-4 0 3 0", "0 1 -4", "0 -3 3 0 -2", "0 -2 0 2", "-2 0 2 0", "3 0 -2 0", "-4 0 -3 0", "0 -3 0 3", "0 3 -3 0", "0 -3 4 -3 0 1 0", "0 3 -2 2 0", "2 0 2", "0 2 0 2 0", "0 3 0 -3", "3 0 -3 4", "0 1 0 1 0", "0 -3 3 -2 0 3", "0 -3 4 -4 0 -3 3 -2", "0 -3 0 2 0", "0 2 -2 0", "0 -3 3 -2", "2 0 -4 0 -3 3", "3 0 -2 3", "0 2 0 -2", "0 2 0 4 0", "-2 0 -2 3 0", "0 1 0 3 0 -2", "-3 3 -3", "0 -3 3 -3", "-3 3 -3 0", "1 0 4", "-4 0 2", "-1 0 -1", "3 0 2", "-3 4 -4", "4 0 3", "-2 0 2", "2 0 3 0", "0 2 -1 0 3", "-3 3 -2", "0 -1 0", "0 3 0", "-1 0 3", "0 3 -2", "-1 0 3 0", "0 1 0", "0 3 0 -1", "-1 0 -1", "3 0 -1", "0 -1 0 3", "-1 1 0", "-1 0 3 -2", "-1 0 -1 0", "0 -1 1 0", "0 -1 0 -1", "0 -1 1", "3 -3 0", "0 1 -1", "0 3 -3", "0 -1 0 -1 0", "0 -3 3", "0 -3 3 0", "0 3 0 3", "1 0 -1", "0 1 -1 0 3", "0 3 0 -1 1 0", "2 -1 0", "1 0 3", "0 3 -2 0", "0 3 -3 0", "0 -1 0 1", "0 2 -1 0", "-1 2 0", "0 1 0 -1", "1 0 -1 0", "0 -1 0 3 0", "0 -1 0 3 -2", "-2 2 0", "2 0 -2", "-1 0 3 -2 3 0", "0 -1 0 -1 0 3", "-1 0 3 -2 3", "-1 0 -1 0 3 -2", "0 2 0", "0 -3 0", "0 -1 2 0", "0 -1 0 -1 1 0 3", "0 -1 0 1 -1 0 3 -2", "1 -1 0 3 -2 3", "2 0 3", "0 3 -3 0 3", "0 -3 3 0 1 0", "1 -1 1 0", "0 3 -2 2 0", "3 0 3", "1 0 -3", "-1 1 0 1", "3 0 1 0 3", "0 -1 0 2 -1 0", "-1 0 -3 3 0", "3 0 1", "3 0 1 0", "0 -2 2", "-1 0 3 0 -1", "0 3 -2 0 -1 0", "3 0 -1 1", "1 -1 0 3 -2", "-1 0 3 -2 0", "0 3 0 -1 1", "3 0 -1 1 0", "-2 -1 0", "-1 0 -1 0 3", "0 -4 0 1 0", "3 0 -1 0", "3 0 -1 0 3", "1 -1 0 3", "1 0 3 0", "0 3 -2 0 1", "0 1 0 -1 0", "0 1 -1 0 3 0", "3 -2 0", "-1 0 1", "1 0 1", "1 -1 0", "0 -1 0", "-1 0 -1", "0 -1 0 -1", "1 -1 0", "0 1 0", "-1 0 3", "2 -1 0", "0 3 0", "0 -1 1", "-1 0 -2", "-2 2 -2", "-1 0 -1 0", "3 -3 0", "0 -2 0", "0 1 -1 0", "-2 0 -1", "0 3 -2", "-2 0 -1 0", "4 -3 0", "0 -1 1 -1 0", "0 -1 0 -1 0", "0 -1 0 3", "-3 0 1", "-1 0 3 0", "3 0 -1", "2 0 3", "0 2 0", "-1 0 -3", "0 -2 3", "0 -1 0 -2", "0 -1 0 -1 1", "0 2 -1", "-1 0 3 -2", "0 1 0 3", "-2 2 -1 0", "2 0 -1", "3 -3 0 1", "-1 0 1 0", "-2 2 0", "3 -2 0 -1 0", "-1 0 2", "0 2 -1 0", "1 0 1", "0 -4 0", "0 4 -3", "0 4 -3 0", "0 -1 0 -3", "0 -3 3 -3 0", "-2 2 -2 0", "-3 0 4", "0 3 -2 0 -1 0", "0 1 0 3 0", "0 3 -3 0", "2 -1 0 2", "-1 0 2 -1", "1 -1 0 -2", "-1 0 1", "3 -2 2", "0 -1 1 0", "-1 0 -2 2", "0 3 0 -1", "-3 0 1 0", "0 -1 0 3 0", "2 -2 0", "0 -3 0", "0 2 0 3", "3 -3 0 1 0", "1 0 -2", "-2 3 0", "-2 0 -2", "2 0 -1 0", "0 -1 0 1", "0 -1 2", "2 0 3 0", "3 0 -2", "0 2 0 -1", "-3 0 2", "-1 0 -2 3", "3 0 -1 1", "3 0 -1 1 -1 0", "0 2 3", "1 -1 0 3", "3 -2 2 -1 0", "-2 2 -2 2", "0 -1 0 -2 2", "-1 0 -1 0 -1", "0 -1 0 -1 1 -1 0", "2 -2 3", "-1 0 -1 0 -2", "-1 0 -2 0", "3 0 1", "0 3 0 1", "-1 0 3 -2 0 -1 0", "0 3 -2 2 -1 0", "0 1 0 -1 0", "3 0 1 0", "2 -1 0 -1", "0 -2 0 -1", "0 1 -1 0 -2 3", "-4 0 1", "0 2 0 -1 0", "-1 0 3 0 -1", "3 0 -1 0", "0 3 0 3", "3 -3 0 2", "-3 0 1 0 1", "0 3 0 -3", "-3 0 3", "4 -3 0 3", "-2 2 -2 0 -2", "2 -2 0 -2 0", "-1 0 -3 3 -3 0", "1 -1 0 -3", "0 -1 0 1 0", "0 -3 -2 3 -3 0", "-2 0 2 0 3 0", "3 0 -2 0", "0 -2 0 1", "0 -1 0 -3 0", "0 3 0 -1 1 -1 0", "-2 2 0 -1", "2 0 -1 1", "3 -2 0 -1 0 -3", "0 3 -3 0 1 0", "0 -3 3 -3 0 1", "0 -2 3 0", "2 -2 0 -2", "-3 0 1 -1 0", "-1 2 0 3", "0 -1 0 -1 1 -1 0 -2 0", "-2 2 -1 0 3", "-2 2 -1 0 3 -2", "2 3 0", "0 -1 0 2", "-1 3 0", "3 0 2", "3 -1 3", "-2 3 0 -1 1", "-2 3 0 -1", "0 -1 0 -1 0 -2", "0 -4 1", "-4 1 0", "0 -1 1 0 -2 0", "0 -2 3 -2 2", "3 -2 2 -1 0 3", "2 -2 3 0 -1", "1 -1 0 -1 0", "1 0 2", "-1 0 -4", "2 -1 0 -1 0", "-1 0 -1 1", "0 3 -2 0 -1 0 -1 0", "1 -1 0 3 -2 0 -1 0 -1", "0 -1 0 -1 0 -1 1", "0 1 0 3 -2", "0 -1 0 -1 1 0", "0 -1 0 3 -2 2 -1 0", "1 0 1 -1 0", "3 -2 0", "3 -2 0 -1", "-2 0 -1 0 3", "0 1 -1", "0 3 0 1 0", "3 0 -3", "2 -2 2", "-2 0 -1 0 -1", "3 -2 0 -1 0 -1", "0 -2 2", "0 3 -2 0", "0 3 -2 0 -1", "1 0 3", "-1 1 0"]) -> (1 "vector (directional transitions)":dbl[][](array[numeric]), 2 "vector (NON directional transitions)":dbl[][](array[numeric]), 3 "vector positions only":dbl[][](array[numeric]))   [LabVIEW 2014]
panel:
  out "Position weights 3":i32[](array[numeric])
  out "averaged position weights 3":dbl[](array[numeric])
  out "Transition weights 2":i32[](array[numeric])
  out "Position weights 2":i32[](array[numeric])
  out "averaged transition weights 2":dbl[](array[numeric])
  out "averaged position weights 2":dbl[](array[numeric])
  out "averaged position weights":dbl[](array[numeric])
  out "averaged transition weights":dbl[](array[numeric])
  out "Position weights":i32[](array[numeric])
  out "Transition weights":i32[](array[numeric])
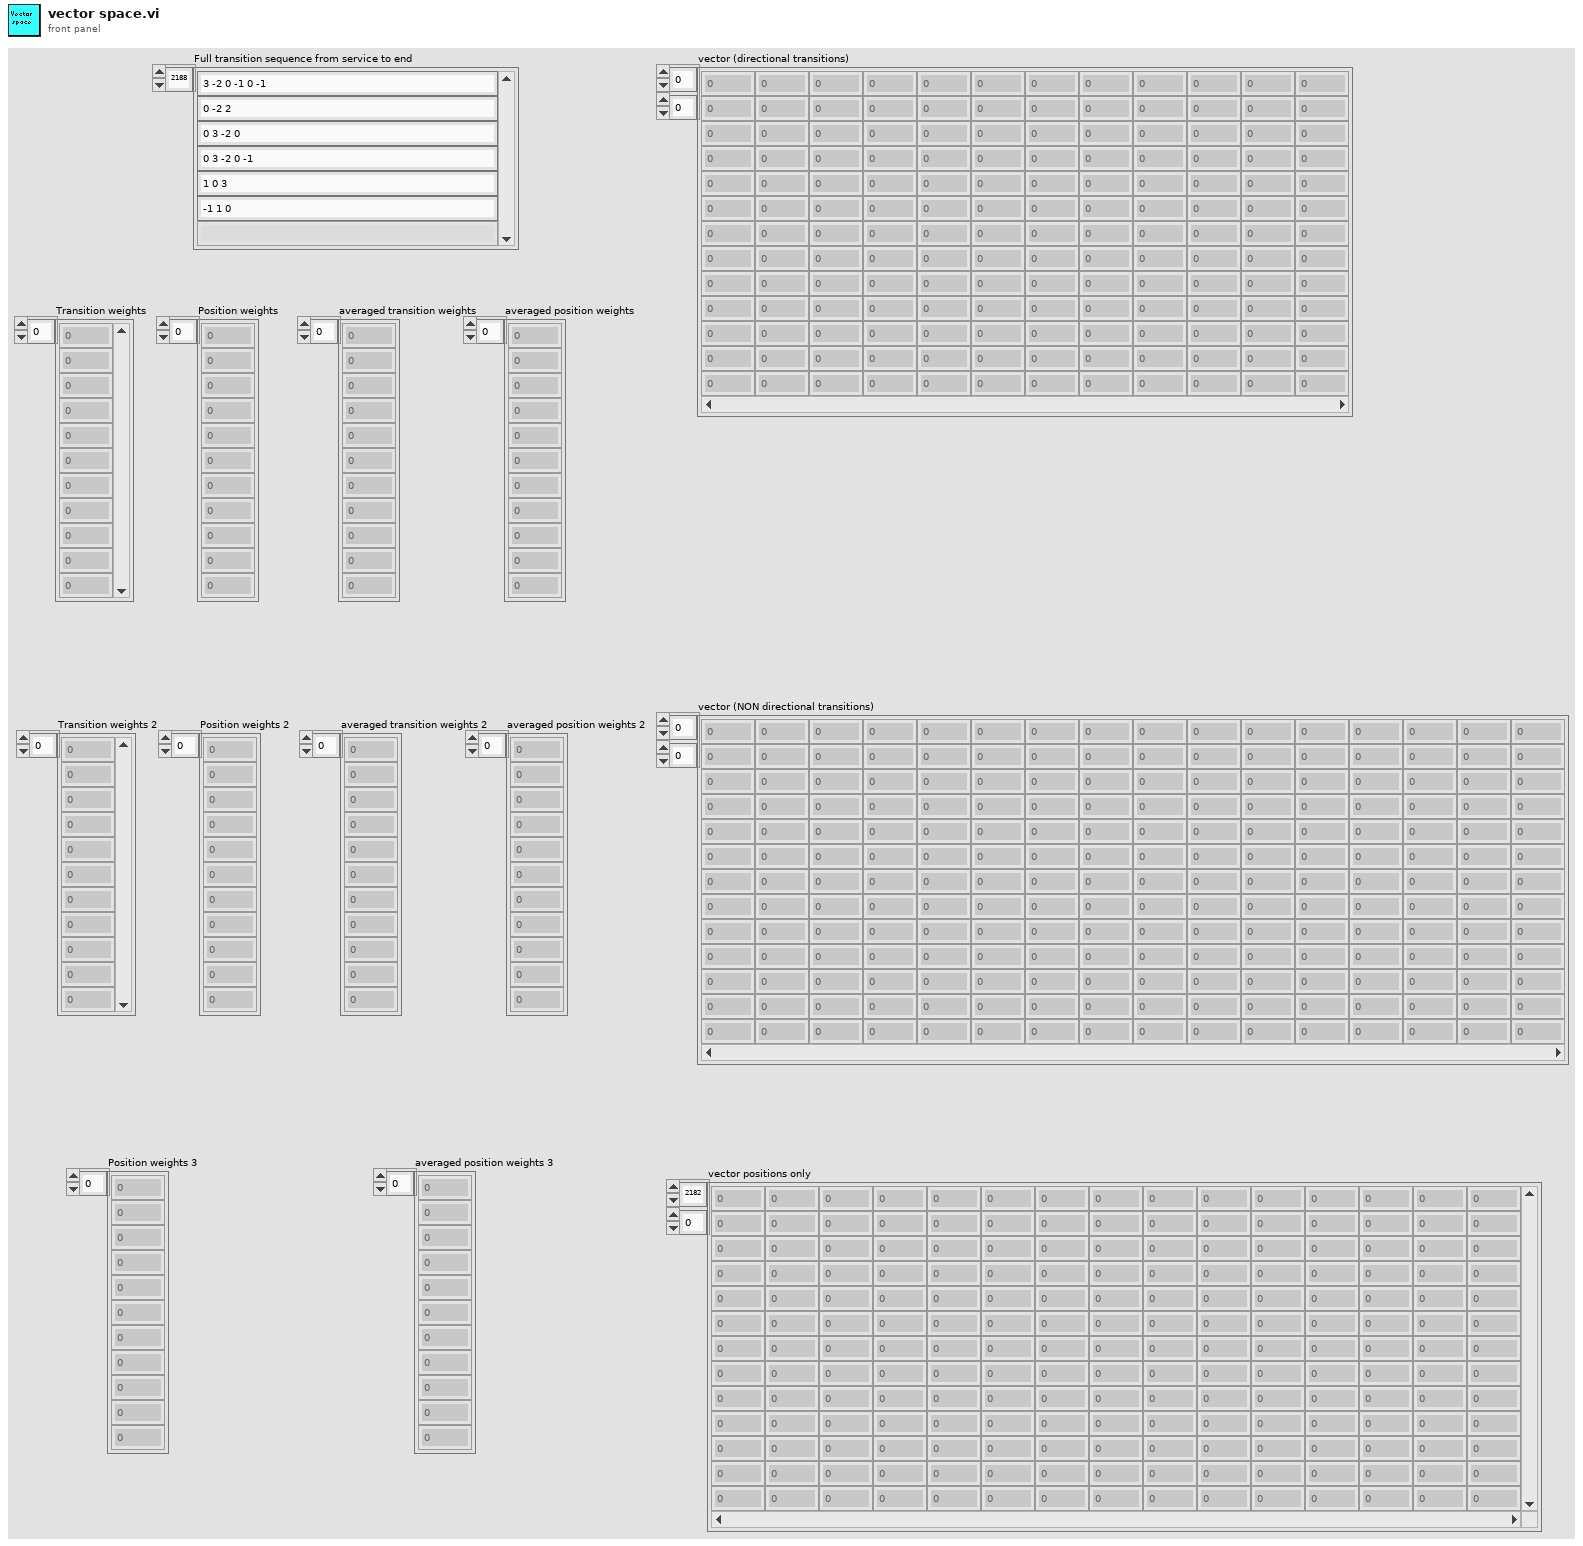
[diagram p1: front panel]
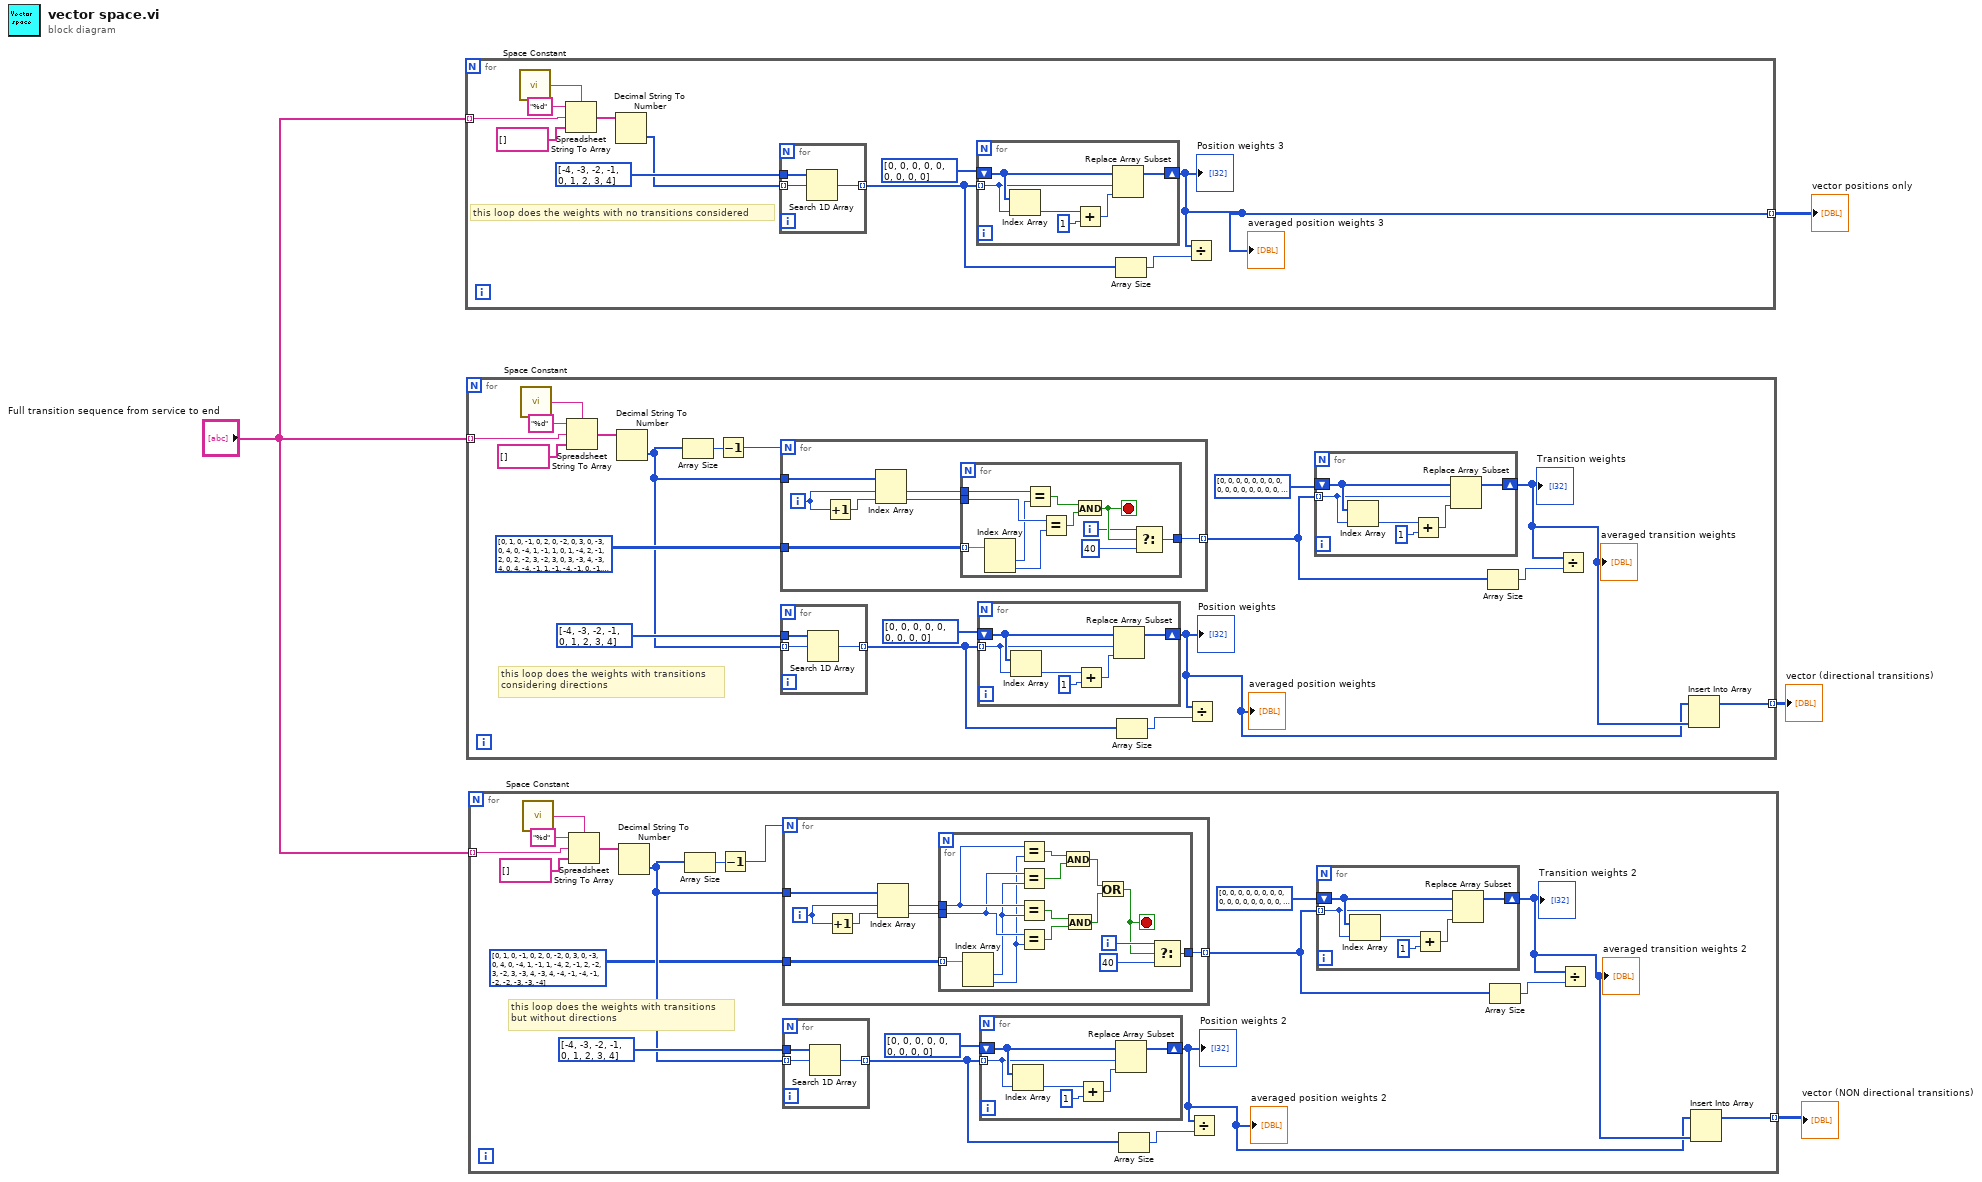
[diagram p0: block diagram]
diagram:
  n1 = for {
    tunnel: "Full transition sequence from service to end" -> [w11] mode=indexing
    tunnel: [w5] -> w1 mode=indexing
    # "this loop does the weights with no transitions considered"
    n2 = call <vilib>:"Space Constant.vi"() -> ("String"=w15:string)
    n3 = Spreadsheet String To Array(delimiter (Tab)=w15, format string="%d", spreadsheet string=w11, array type (2D Dbl)=string[] []) -> (array=w12:string[])
    n4 = Decimal String To Number(string=w12) -> (number=w9:i32[])  [unwired: 2 in, 1 out]
    n5 = for {
      tunnel: i32[] [-4, -3, -2, -1, 0, 1, 2, 3, 4] ("deleted portion") -> [w24]
      tunnel: w9 -> [w23] mode=indexing
      tunnel: [w22] -> w6 mode=indexing
      n6 = Search 1D Array(1D array=w24, element=w23) -> (index of element=w22:i32)  [unwired: 1 in]
    }
    n7 = for {
      tunnel: w6 -> [w18] mode=indexing
      shift-right: [w16] -> w5
      shift-left: i32[] [0, 0, 0, 0, 0, 0, 0, 0, 0] ("deleted portion") -> [w19]
      n8 = Index Array(array=w19, index=w18) -> (element=w21:i32)
      n9 = Add(x=w21, y=1) -> (x+y=w17:i32)
      n10 = Replace Array Subset(array=w19, new element=w17, index=w18) -> (w16:i32[])
    }
    "Position weights 3" <- w5
    "averaged position weights 3" <- w5
    n11 = Array Size(array=w6) -> (size(s)=w7:i32)
    n12 = Divide(x=w5, y=w7) -> ()  [unwired: 1 out]
  }
  "vector positions only" <- w1
  n13 = for {
    tunnel: "Full transition sequence from service to end" -> [w37] mode=indexing
    tunnel: [w27] -> w4 mode=indexing
    # "this loop does the weights with transitions\nconsidering directions"
    n14 = call <vilib>:"Space Constant.vi"() -> ("String"=w43:string)
    n15 = Spreadsheet String To Array(delimiter (Tab)=w43, format string="%d", spreadsheet string=w37, array type (2D Dbl)=string[] []) -> (array=w40:string[])
    n16 = Decimal String To Number(string=w40) -> (number=w33:i32[])  [unwired: 2 in, 1 out]
    n17 = Array Size(array=w33) -> (size(s)=w39:i32)
    n18 = Decrement(x=w39) -> (x-1=w38:i32)
    n19 = for {
      N: w38 -> [_]
      tunnel: w33 -> [w64]
      tunnel: i32[][] [[0, 1], [0, -1], [0, 2], [0, -2], [0, 3], [0, -3], [0, 4], [0, -4], [1, -1], [1, 0], [1, -4], [2, -1], [2, 0], [2, -2], [3, -2], [3, 0], [3, -3], [4, -3], [4, 0], [4, -4], [-1, 1], [-1, -4], [-1, 0], [-1, -2], [-1, 2], [-2, 2], [-2, -1], [-2, 0], [-2, -3], [-2, 3], [-3, 3], [-3, -2], [-3, 0], [-3, -4], [-3, 4], [-4, 4], [-4, -3], [-4, 0], [-4, -1], [-4, 1]] -> [w65]
      tunnel: [w59] -> w31 mode=indexing
      i -> [w63]
      n20 = Increment(x=w63) -> (x+1=w62:i32)
      n21 = Index Array(array=w64, index #1=w63, index #2=w62) -> (element #1=w61:i32, element #2=w60:i32)
      n22 = for {
        tunnel: w65 -> [w76] mode=indexing
        tunnel: w61 -> [w75]
        tunnel: w60 -> [w74]
        tunnel: [w66] -> w59
        i -> [w67]
        stop <- w69 stop-if-true
        n23 = Index Array(array=w76) -> (element #1=w73:i32, element #2=w72:i32)  [unwired: 2 in]
        n24 = Equal?(x=w75, y=w73) -> (x = y?=w71:bool)
        n25 = Equal?(x=w74, y=w72) -> (x = y?=w70:bool)
        n26 = And(x=w71, y=w70) -> (x .and. y?=w69:bool)
        n27 = Select(t=w67, s=w69, f=40) -> (s? t:f=w66:i32)
      }
    }
    n28 = for {
      tunnel: i32[] [-4, -3, -2, -1, 0, 1, 2, 3, 4] ("deleted portion") -> [w52]
      tunnel: w33 -> [w51] mode=indexing
      tunnel: [w50] -> w28 mode=indexing
      n29 = Search 1D Array(1D array=w52, element=w51) -> (index of element=w50:i32)  [unwired: 1 in]
    }
    n30 = for {
      tunnel: w28 -> [w46] mode=indexing
      shift-right: [w44] -> w25
      shift-left: i32[] [0, 0, 0, 0, 0, 0, 0, 0, 0] ("deleted portion") -> [w47]
      n31 = Index Array(array=w47, index=w46) -> (element=w49:i32)
      n32 = Add(x=w49, y=1) -> (x+y=w45:i32)
      n33 = Replace Array Subset(array=w47, new element=w45, index=w46) -> (w44:i32[])
    }
    "Position weights" <- w25
    "averaged position weights" <- w25
    n34 = Array Size(array=w28) -> (size(s)=w29:i32)
    n35 = Divide(x=w25, y=w29) -> ()  [unwired: 1 out]
    n36 = for {
      tunnel: w31 -> [w55] mode=indexing
      shift-right: [w53] -> w26
      shift-left: i32[] [0, 0, 0, 0, 0, 0, 0, 0, 0, 0, 0, 0, 0, 0, 0, 0, 0, 0, 0, 0, 0, 0, 0, 0, 0, 0, 0, 0, 0, 0, 0, 0, 0, 0, 0, 0, 0, 0, 0, 0] ("deleted portion") -> [w56]
      n37 = Index Array(array=w56, index=w55) -> (element=w58:i32)
      n38 = Add(x=w58, y=1) -> (x+y=w54:i32)
      n39 = Replace Array Subset(array=w56, new element=w54, index=w55) -> (w53:i32[])
    }
    "Transition weights" <- w26
    "averaged transition weights" <- w26
    n40 = Array Size(array=w31) -> (size(s)=w30:i32)
    n41 = Divide(x=w26, y=w30) -> ()  [unwired: 1 out]
    n42 = Insert Into Array(array=w25, new element=w26) -> (w27:i32[])  [unwired: 1 in]
  }
  "vector (directional transitions)" <- w4
  n43 = for {
    tunnel: "Full transition sequence from service to end" -> [w89] mode=indexing
    tunnel: [w81] -> w3 mode=indexing
    # "this loop does the weights with transitions\nbut without directions"
    n44 = call <vilib>:"Space Constant.vi"() -> ("String"=w95:string)
    n45 = Spreadsheet String To Array(delimiter (Tab)=w95, format string="%d", spreadsheet string=w89, array type (2D Dbl)=string[] []) -> (array=w92:string[])
    n46 = Decimal String To Number(string=w92) -> (number=w87:i32[])  [unwired: 2 in, 1 out]
    n47 = Array Size(array=w87) -> (size(s)=w91:i32)
    n48 = Decrement(x=w91) -> (x-1=w90:i32)
    n49 = for {
      N: w90 -> [_]
      tunnel: w87 -> [w116]
      tunnel: i32[][] [[0, 1], [0, -1], [0, 2], [0, -2], [0, 3], [0, -3], [0, 4], [0, -4], [1, -1], [1, -4], [2, -1], [2, -2], [3, -2], [3, -3], [4, -3], [4, -4], [-1, -4], [-1, -2], [-2, -3], [-3, -4]] -> [w117]
      tunnel: [w111] -> w85 mode=indexing
      i -> [w115]
      n50 = Increment(x=w115) -> (x+1=w114:i32)
      n51 = Index Array(array=w116, index #1=w115, index #2=w114) -> (element #1=w113:i32, element #2=w112:i32)
      n52 = for {
        tunnel: w117 -> [w132] mode=indexing
        tunnel: w113 -> [w126]
        tunnel: w112 -> [w125]
        tunnel: [w127] -> w111
        i -> [w128]
        stop <- w118 stop-if-true
        n53 = Index Array(array=w132) -> (element #1=w124:i32, element #2=w123:i32)  [unwired: 2 in]
        n54 = Equal?(x=w126, y=w123) -> (x = y?=w122:bool)
        n55 = Equal?(x=w125, y=w124) -> (x = y?=w121:bool)
        n56 = Equal?(x=w126, y=w124) -> (x = y?=w131:bool)
        n57 = Equal?(x=w125, y=w123) -> (x = y?=w130:bool)
        n58 = And(x=w122, y=w121) -> (x .and. y?=w120:bool)
        n59 = And(x=w131, y=w130) -> (x .and. y?=w119:bool)
        n60 = Or(x=w120, y=w119) -> (x .or. y?=w118:bool)
        n61 = Select(t=w128, s=w118, f=40) -> (s? t:f=w127:i32)
      }
    }
    n62 = for {
      tunnel: i32[] [-4, -3, -2, -1, 0, 1, 2, 3, 4] ("deleted portion") -> [w104]
      tunnel: w87 -> [w103] mode=indexing
      tunnel: [w102] -> w82 mode=indexing
      n63 = Search 1D Array(1D array=w104, element=w103) -> (index of element=w102:i32)  [unwired: 1 in]
    }
    n64 = for {
      tunnel: w82 -> [w98] mode=indexing
      shift-right: [w96] -> w77
      shift-left: i32[] [0, 0, 0, 0, 0, 0, 0, 0, 0] ("deleted portion") -> [w99]
      n65 = Index Array(array=w99, index=w98) -> (element=w101:i32)
      n66 = Add(x=w101, y=1) -> (x+y=w97:i32)
      n67 = Replace Array Subset(array=w99, new element=w97, index=w98) -> (w96:i32[])
    }
    "Position weights 2" <- w77
    "averaged position weights 2" <- w77
    n68 = Array Size(array=w82) -> (size(s)=w83:i32)
    n69 = Divide(x=w77, y=w83) -> ()  [unwired: 1 out]
    n70 = for {
      tunnel: w85 -> [w107] mode=indexing
      shift-right: [w105] -> w78
      shift-left: i32[] [0, 0, 0, 0, 0, 0, 0, 0, 0, 0, 0, 0, 0, 0, 0, 0, 0, 0, 0, 0] ("deleted portion") -> [w108]
      n71 = Index Array(array=w108, index=w107) -> (element=w110:i32)
      n72 = Add(x=w110, y=1) -> (x+y=w106:i32)
      n73 = Replace Array Subset(array=w108, new element=w106, index=w107) -> (w105:i32[])
    }
    "Transition weights 2" <- w78
    "averaged transition weights 2" <- w78
    n74 = Array Size(array=w85) -> (size(s)=w84:i32)
    n75 = Divide(x=w78, y=w84) -> ()  [unwired: 1 out]
    n76 = Insert Into Array(array=w77, new element=w78) -> (w81:i32[])  [unwired: 1 in]
  }
  "vector (NON directional transitions)" <- w3
